vi "LEBITplc.UpdateResistorChain.vi"(0 "i ref in":refnum<vi>, 2 "Value 1":dbl, 3 "Value 2":dbl, 4 "index in":i32, 5 "error out in":errorcluster, 8 "Enum":enum16{"DCS", "MFDCS"}(ring)) -> (14 "i ref out":refnum<vi>, 19 "error out":errorcluster)   [LabVIEW 2014, in "LEBITplc.lvlib"]
uses:
  LEBITplc.lvlib
  CSlibraries-extern/DimLVEvent/LVDimInterface/LVDimInterface.lvlib
panel:
  out "index out":i32
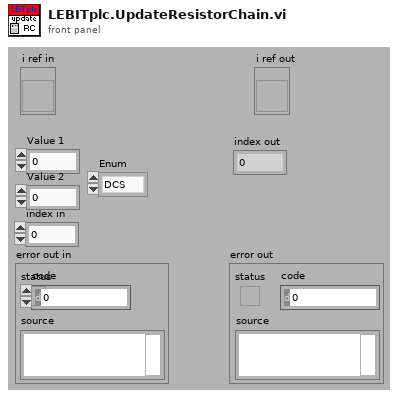
[diagram p1: front panel]
types:
  T1 = typedef "LEBITplc.lvlib/LEBITplc.i attribute.ctl" = cluster{"LLFLocation":string, "SetFileLocation":string, "nickNames":string[], "setValuePLCServiceID":i32[], "GUIServiceID":i32[], "monValuePLC":string[], "SetValueServiceID":i32[], "MonValueServiceID":i32[], "SetValue":dbl[][], "SetValueMin":dbl[], "SetValueMax":dbl[], "SetValueInfoServiceID":i32[], "GUINames":string[], "ListOfBases":string[], "Scale":dbl[], "Offset":dbl[], "setValuePLC":string[], "BaseName":string[], "ScaleServiceID":i32[], "OffsetServiceID":i32[], "AllPLCValues":string[], "CondSpecialArray":string[][], "CondSpecialIndex":i32[], "CondSpecialMonValue":dbl[], "RecentlyChanged":i32[], "SetFileLocationID":i32, "Dependent-Monitors":string[][], "LastLoadedFiles":string[], "IonGuideCalibLocation":string, "Monitor Dependent":string[], "Special":string[], "PLC?":bool[], "Start Date":string, "ListOfBasesServiceID":i32, "SETRA VISA resource":refnum<visa-resource-name>}
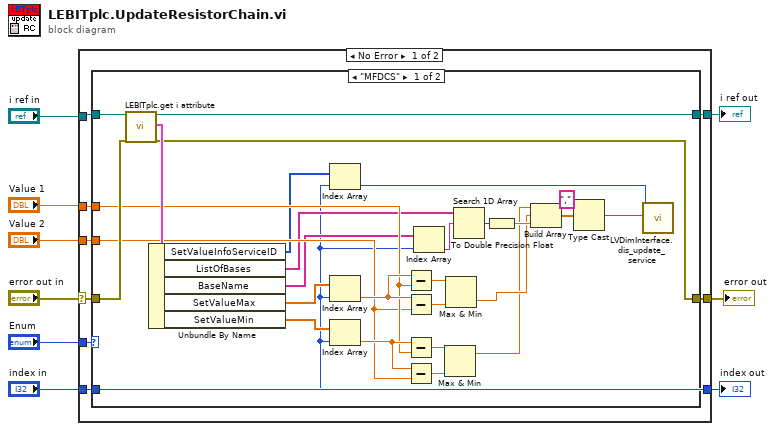
[diagram p0: block diagram]
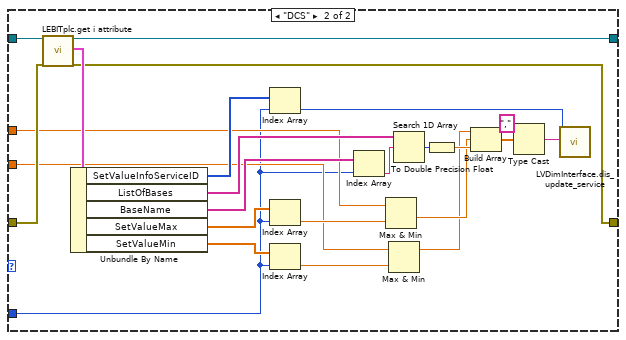
[diagram p2: hidden frame]
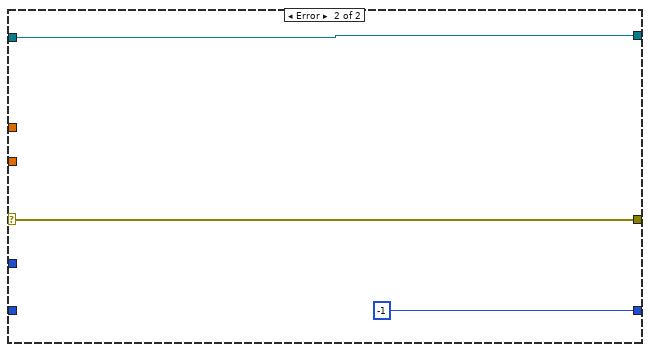
[diagram p3: hidden frame]
diagram:
  n1 = case shown="No Error" "error out in" {
    selector: "error out in" -> [w16 w71]
    tunnel: "i ref in" -> [w17 w72]
    tunnel: [w15 w72] -> w6
    tunnel: [w14 w71] -> w7
    tunnel: [w11 -1 ("index of element")] -> w5
    tunnel: "index in" -> [w11 _]
    tunnel: "Value 1" -> [w13 _]
    tunnel: "Value 2" -> [w12 _]
    tunnel: "Enum" -> [w10 _]
    frame No Error {
      n2 = case shown="\"MFDCS\"" w10 {
        tunnel: w17 -> [w41 w69]
        tunnel: w16 -> [w40 w68]
        tunnel: [w19 w47] -> w15
        tunnel: [w18 w46] -> w14
        tunnel: w13 -> [w34 w51]
        tunnel: w12 -> [w33 w49]
        tunnel: w11 -> [w20 w48]
        frame "MFDCS" {
          n3 = call "LEBITplc.get i attribute.vi"("i ref in"=w41, "error in (no error)"=w40) -> ("i ref out"=w19:refnum<vi>, "i attribute"=w35:T1, "error out"=w18:errorcluster)  [unwired: 15 in]
          n4 = Unbundle By Name(w35) -> ("SetValueInfoServiceID"=w24:i32[], "ListOfBases"=w25:string[], "BaseName"=w30:string[], "SetValueMax"=w37:dbl[], "SetValueMin"=w36:dbl[])
          n5 = Index Array(array=w24, index=w20) -> (element=w23:i32)
          n6 = Index Array(array=w37, index=w20) -> (element=w45:dbl)
          n7 = Index Array(array=w36, index=w20) -> (element=w44:dbl)
          n8 = Subtract(x=w45, y=w34) -> (x-y=w42:dbl)
          n9 = Subtract(x=w45, y=w33) -> (x-y=w43:dbl)
          n10 = Subtract(x=w44, y=w34) -> (x-y=w39:dbl)
          n11 = Subtract(x=w44, y=w33) -> (x-y=w38:dbl)
          n12 = Index Array(array=w30, index=w20) -> (element=w32:string)
          n13 = Max & Min(x=w39, y=w38) -> (max(x,y)=w21:dbl)  [unwired: 1 out]
          n14 = Max & Min(x=w42, y=w43) -> (min(x,y)=w22:dbl)  [unwired: 1 out]
          n15 = Search 1D Array(1D array=w25, element=w32) -> (index of element=w31:i32)  [unwired: 1 in]
          n16 = To Double Precision Float(number=w31) -> (double precision float=w26:dbl)
          n17 = Build Array(w21, w22, w26) -> (w27:dbl[])
          n18 = Type Cast(type="," ("regular expression"), x=w27) -> (*(type *) &x=w29:string)
          n19 = call "LVDimInterface.dis_update_service.vi"("my_serviceID"=w23, "data"=w29) -> ()  [unwired: 15 in, 3 out]
        }
        frame "DCS" {
          n20 = call "LEBITplc.get i attribute.vi"("i ref in"=w69, "error in (no error)"=w68) -> ("i ref out"=w47:refnum<vi>, "i attribute"=w65:T1, "error out"=w46:errorcluster)  [unwired: 15 in]
          n21 = Unbundle By Name(w65) -> ("SetValueInfoServiceID"=w56:i32[], "ListOfBases"=w57:string[], "BaseName"=w62:string[], "SetValueMax"=w67:dbl[], "SetValueMin"=w66:dbl[])
          n22 = Index Array(array=w56, index=w48) -> (element=w55:i32)
          n23 = Index Array(array=w67, index=w48) -> (element=w50:dbl)
          n24 = Index Array(array=w66, index=w48) -> (element=w52:dbl)
          n25 = Index Array(array=w62, index=w48) -> (element=w64:string)
          n26 = Max & Min(x=w51, y=w50) -> (min(x,y)=w54:dbl)  [unwired: 1 out]
          n27 = Max & Min(x=w49, y=w52) -> (max(x,y)=w53:dbl)  [unwired: 1 out]
          n28 = Search 1D Array(1D array=w57, element=w64) -> (index of element=w63:i32)  [unwired: 1 in]
          n29 = To Double Precision Float(number=w63) -> (double precision float=w58:dbl)
          n30 = Build Array(w53, w54, w58) -> (w59:dbl[])
          n31 = Type Cast(type="," ("regular expression"), x=w59) -> (*(type *) &x=w61:string)
          n32 = call "LVDimInterface.dis_update_service.vi"("my_serviceID"=w55, "data"=w61) -> ()  [unwired: 15 in, 3 out]
        }
      }
    }
    frame Error {
    }
  }
  "error out" <- w7
  "i ref out" <- w6
  "index out" <- w5
